vi "compress_exe.vi"(8 "error in (no error)":errorcluster, 10 "files_to_add":path, 11 "archive_path in":path) -> (0 "error out":errorcluster, 3 "archive_path out":path)   [LabVIEW 2015, in "lv-bin-7zip.lvlib" / "v1.lvlib"]
uses:
  v1.lvlib
  lv-bin-7zip.lvlib
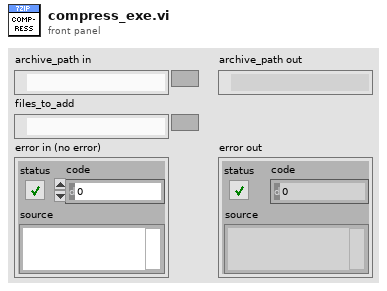
[diagram p1: front panel]
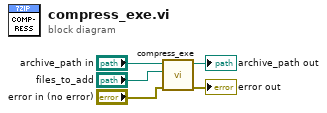
[diagram p0: block diagram]
diagram:
  n1 = call "compress_exe.vi"("error in (no error)"="error in (no error)", "files_to_add"="files_to_add", "archive_path in"="archive_path in") -> ("error out"=→"error out":errorcluster, "archive_path out"=→"archive_path out":path)  [unwired: 7 in]
